vi "create.vi"(8 "error in":errorcluster, 9 "dt":dbl=5e-08 caption="dt (s)" format="%#_6p", 10 "output_settings":T2={"phase_corr"=-0.25, "ramp ends"=TRUE, "ramp time"=1e-05, "add func"=TRUE, "f(x, t)"="-3 * exp(-(t-8E-5)^2/(2 * (1E-6^2)))"} {"ramp time" format="%#_6p"}, 11 "beam settings":T3={"initial velocity"=2000.0, "cell length"=0.025, "electrodes/ cell"=5, "stages"=[{"final vel. (m/s)"=0.0, "distance (m)"=0.05, "hold (s)"=1e-05}, {"final vel. (m/s)"=1250.0, "distance (m)"=0.025, "hold (s)"=0.0}]} {"cell length" format="%#_6p"; "initial velocity" format="%#_6p"; "stages"."hold (s)" format="%#_6p"; "stages"."distance (m)" format="%#_6p"; "stages"."final vel. (m/s)" format="%#_6p"}) -> (0 "error out":errorcluster, 1 "correction":waveform(dbl)[](graph), 2 "electrodes":waveform(dbl)[](graph)=[{"t0"=timestamp(0 s since 1904-01-01), "dt"=5e-08, "Y"=array[2000 elements]}, {"t0"=timestamp(0 s since 1904-01-01), "dt"=5e-08, "Y"=array[2000 elements]}, {"t0"=timestamp(0 s since 1904-01-01), "dt"=5e-08, "Y"=array[2000 elements]}, {"t0"=timestamp(0 s since 1904-01-01), "dt"=5e-08, "Y"=array[2000 elements]}, {"t0"=timestamp(0 s since 1904-01-01), "dt"=5e-08, "Y"=array[2000 elements]}], 3 "wf":T1)   [LabVIEW 2013, in "wf_tools.lvlib"]
uses:
  wf_tools.lvlib
  wf.ctl
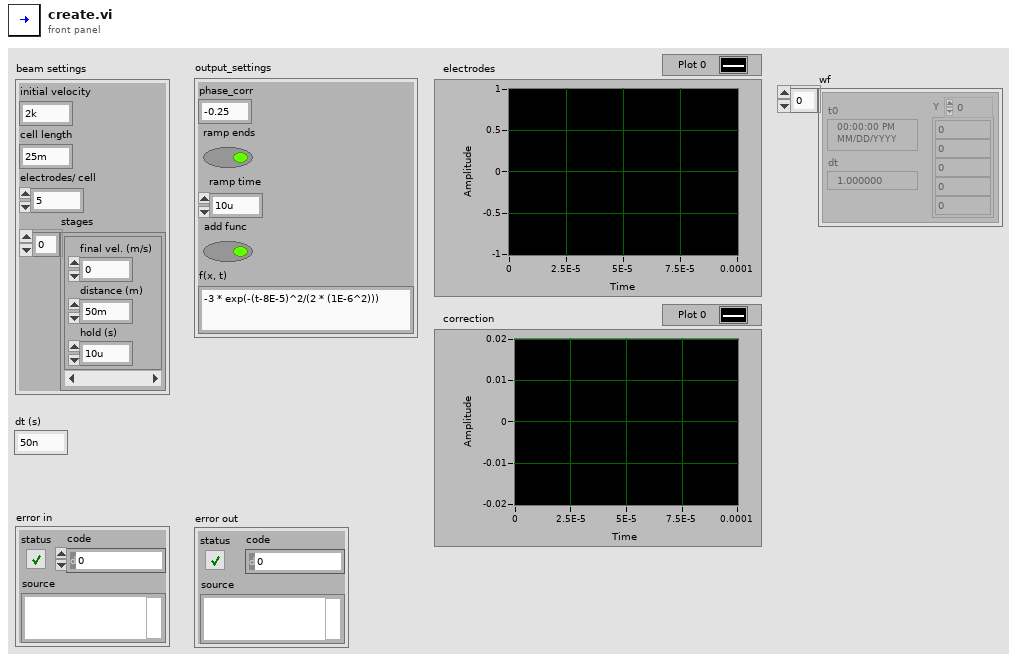
[diagram p1: front panel]
types:
  T1 = typedef "wf_tools.lvlib/wf.ctl" = waveform(dbl)[]
  T2 = cluster{"phase_corr":dbl, "ramp ends":bool, "ramp time":dbl, "add func":bool, "f(x, t)":string}
  T3 = cluster{"initial velocity":dbl, "cell length":dbl, "electrodes/ cell":i32, "stages":cluster{"final vel. (m/s)":dbl, "distance (m)":dbl, "hold (s)":dbl}[]}
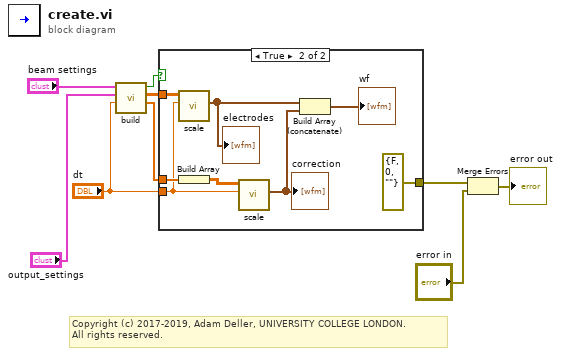
[diagram p0: block diagram]
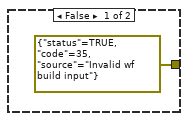
[diagram p2: hidden frame]
diagram:
  # "Copyright (c) 2017-2019, Adam Deller, UNIVERSITY COLLEGE LONDON.\nAll rights reserved."
  n1 = call "build.vi"("dt"="dt", "output_settings"="output_settings", "beam settings"="beam settings") -> ("corr_wf"=w7:dbl[], "el_wf"=w8:dbl[][], "valid"=w5:bool)  [unwired: 4 in, 2 out]
  n2 = case shown="True" w5 {
    tunnel: w8 -> [_ w18]
    tunnel: w7 -> [_ w17]
    tunnel: "dt" -> [_ w15]
    tunnel: [errorcluster {"status"=TRUE, "code"=35, "source"="Invalid wf build input"} ("error constant") errorcluster {"status"=FALSE, "code"=0, "source"=""} ("error constant")] -> w3
    frame False {
    }
    frame True {
      n3 = call "scale.vi"("dt"=w15, "waveforms"=w18) -> ("el"=w13:waveform(dbl)[])  [unwired: 9 in]
      "electrodes" <- w13
      n4 = Build Array(w17) -> (w16:dbl[][])
      n5 = call "scale.vi"("dt"=w15, "waveforms"=w16) -> ("el"=w12:waveform(dbl)[])  [unwired: 9 in]
      "correction" <- w12
      n6 = Build Array (concatenate)(w13, w12) -> (→"wf":waveform(dbl)[])
    }
  }
  n7 = Merge Errors(w3, "error in") -> (→"error out":errorcluster)
